vi "dfd_Validate Fs.vi"(6 "fs [Hz]":dbl=1.0 format="%.2f", 8 "error in (no error)":errorcluster) -> (0 "error out":errorcluster, 4 "dup fs [Hz]":dbl format="%.2f")   [LabVIEW 2017, in "NI_DigFilterLicensed.lvlib"]
uses:
  <vilib>/addons/Digital Filter Design/NI_DigFilterLicensed.lvlib
  <vilib>/addons/Digital Filter Design/_Misc.llb/dfd_Error Handlers (Single).vi
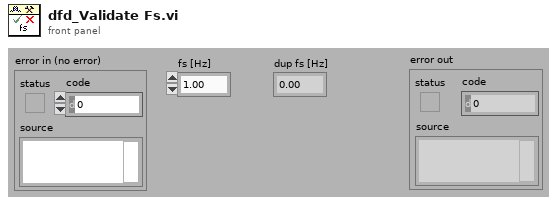
[diagram p1: front panel]
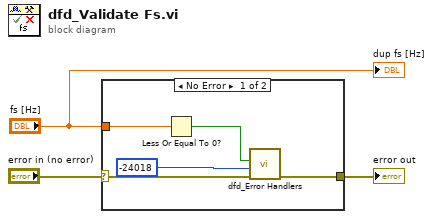
[diagram p0: block diagram]
diagram:
  n1 = case shown="No Error" "error in (no error)" {
    selector: "error in (no error)" -> [w5 w9]
    tunnel: "fs [Hz]" -> [w8 _]
    tunnel: [w4 w9] -> w1
    frame No Error {
      n2 = Less Or Equal To 0?(x=w8) -> (x <= 0?=w6:bool)
      n3 = call-poly <vilib>:"dfd_Error Handlers.vi"("error in (no error)"=w5, "error code"=-24018 ("ERR_FS_LE_ZERO"), "condition failed?"=w6) -> ("error out"=w4:errorcluster)  [unwired: 8 out]
    }
    frame Error {
    }
  }
  "error out" <- w1
  "dup fs [Hz]" <- "fs [Hz]"
